vi "MCCPMTInitialize.vi"(8 "error in (no error)":errorcluster, 10 "PMTs":T1={"PMT1"="Dev0/Ao0", "PMT2"="Dev0/Ao1", "PMT3"="Dev0/Ao1"}, 11 "MCCPMT in":refnum<class "MCCPMT.lvclass">) -> (0 "error out":errorcluster, 3 "MCCPMT out":refnum<class "MCCPMT.lvclass">)   [LabVIEW 2012, in "MCCPMT.lvclass"]
uses:
  classes/MCCPMT.lvclass
  typedefs/PMTs.ctl
  classes/MCCPMT.lvclass/MCCPMT.ctl
  <vilib>/ULx/Create Channel.llb/ULx Create Channel (AO-Voltage-Basic).vi
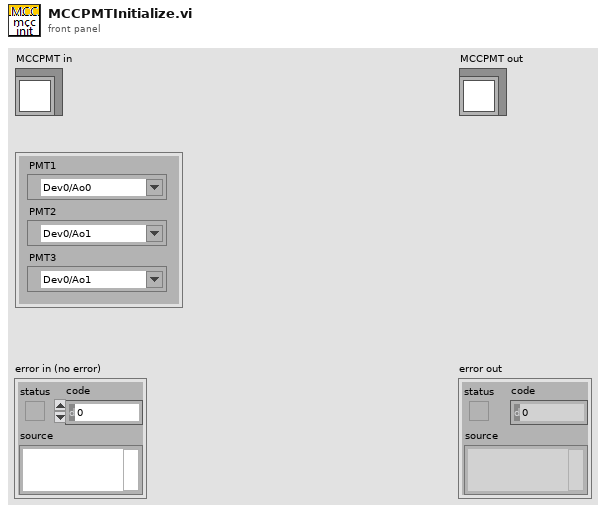
[diagram p1: front panel]
types:
  T1 = typedef "PMTs.ctl" = cluster{"PMT1":refnum<k21>, "PMT2":refnum<k21>, "PMT3":refnum<k21>}
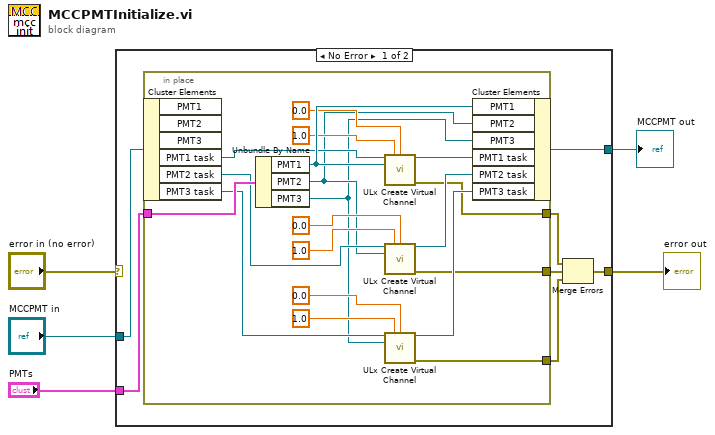
[diagram p0: block diagram]
diagram:
  n1 = case shown="No Error" "error in (no error)" {
    selector: "error in (no error)" -> [_ w33]
    tunnel: [w9 w33] -> w4
    tunnel: [w11 w32] -> w2
    tunnel: "MCCPMT in" -> [w12 w32]
    tunnel: "PMTs" -> [w10 _]
    frame No Error {
      n2 = in-place {
        in-place-border: w10 -> [w29]
        in-place-border: [w15] -> w8
        in-place-border: [w14] -> w7
        in-place-border: [w13] -> w6
        n3 = in-place-cluster #1(w12) -> ("PMT1 task"=w22:refnum<k24>, "PMT2 task"=w23:refnum<k24>, "PMT3 task"=w18:refnum<k24>)  [unwired: 3 out]
        n4 = Unbundle By Name(w29) -> ("PMT1"=w28:refnum<k21>, "PMT2"=w21:refnum<k21>, "PMT3"=w16:refnum<k21>)
        n5 = call-poly <vilib>:"ULx Create Virtual Channel.vi"("task in"=w22, "maximum value"=1.0, "minimum value"=0.0, "physical channels"=w28) -> ("task out"=w31:refnum<k24>, "error out"=w15:errorcluster)  [unwired: 10 in]
        n6 = call-poly <vilib>:"ULx Create Virtual Channel.vi"("task in"=w23, "maximum value"=1.0, "minimum value"=0.0, "physical channels"=w21) -> ("task out"=w30:refnum<k24>, "error out"=w14:errorcluster)  [unwired: 10 in]
        n7 = call-poly <vilib>:"ULx Create Virtual Channel.vi"("task in"=w18, "maximum value"=1.0, "minimum value"=0.0, "physical channels"=w16) -> ("task out"=w17:refnum<k24>, "error out"=w13:errorcluster)  [unwired: 10 in]
        n8 = in-place-cluster #1("PMT1"=w28, "PMT2"=w21, "PMT3"=w16, "PMT1 task"=w31, "PMT2 task"=w30, "PMT3 task"=w17) -> (w11:refnum<class "MCCPMT.lvclass">)
      }
      n9 = Merge Errors(w8, w7, w6) -> (w9:errorcluster)
    }
    frame Error {
    }
  }
  "error out" <- w4
  "MCCPMT out" <- w2
